vi "random sample matlab.vi"(6 "AOM delta":dbl, 7 "INJ delta":dbl, 8 "AOM end":dbl=1.0, 9 "AOM start":dbl, 10 "INJ end":dbl=1.0, 11 "INJ start":dbl) -> (1 "No. of parameters":i32, 3 "Shuffled Parameters":dbl[][](array[numeric]))   [LabVIEW 2014]
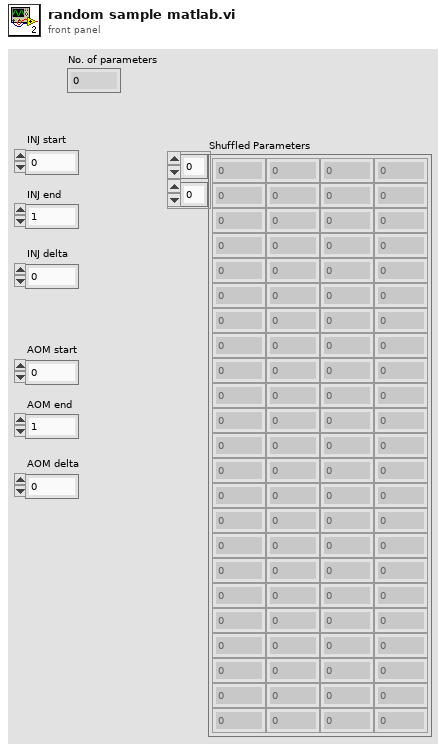
[diagram p1: front panel]
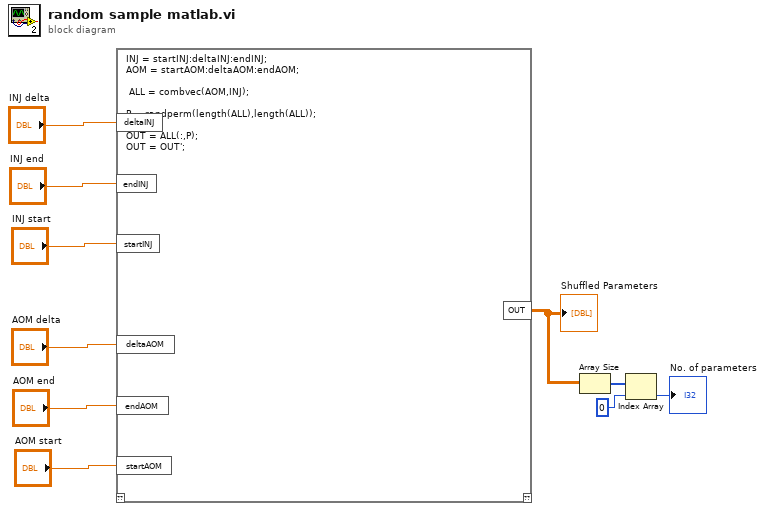
[diagram p0: block diagram]
diagram:
  n1 = script code="INJ = startINJ:deltaINJ:endINJ;\nAOM = startAOM:deltaAOM:endAOM;\n\n ALL = combvec(AOM,INJ);\n\nP = randperm(length(ALL),length(ALL));\n\nOUT = ALL(:,P);\nOUT = OUT';"("deltaINJ"="INJ delta", "endINJ"="INJ end", "startINJ"="INJ start", "deltaAOM"="AOM delta", "endAOM"="AOM end", "startAOM"="AOM start") -> ("OUT"=w4:dbl[][])  [unwired: 1 in, 1 out]
  "Shuffled Parameters" <- w4
  n2 = Array Size(array=w4) -> (size(s)=w3:i32[])
  n3 = Index Array(array=w3, index=0) -> (element=→"No. of parameters":i32)
